vi "Read Variable (Boolean).vi"(8 "error in":errorcluster, 10 "variable name":string, 11 "particle reference in":T1) -> (0 "error out":errorcluster, 2 "value":bool, 3 "particle reference out":T1)   [LabVIEW 2013, in "Particle API.lvlib"]
doc: "Reads Spark registered variables and converts them to the relevant type (bool)."
uses:
  Particle API.lvlib
  Controls/Particle Reference.ctl
  <vilib>/httpClient/ClientHandle.ctl
  Controls/Device Query JSON.ctl
  <vilib>/httpClient/LabVIEWHTTPClient.lvlib
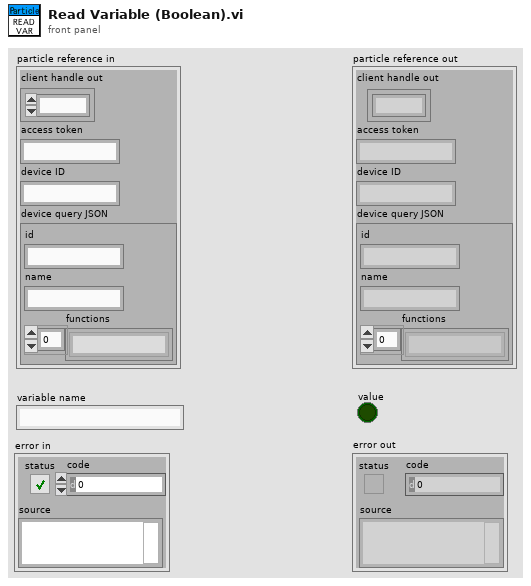
[diagram p1: front panel]
types:
  T1 = typedef "Particle API.lvlib/Particle Reference.ctl" = cluster{"client handle out":T2, "access token":string, "device ID":string, "device query JSON":T3}
  T2 = typedef "LabVIEWHTTPClient.lvlib/ClientHandle.ctl" = refnum<k1>
  T3 = typedef "Particle API.lvlib/Device Query JSON.ctl" = cluster{"id":string, "name":string, "functions":string[]}
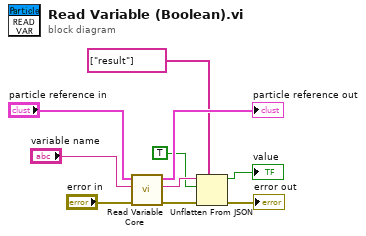
[diagram p0: block diagram]
diagram:
  n1 = call "Read Variable Core.vi"("error in"="error in", "variable name"="variable name", "particle reference in"="particle reference in") -> ("error out"=w5:errorcluster, "variable response"=w3:string, "particle reference out"=→"particle reference out":T1)  [unwired: 6 in]
  n2 = Unflatten From JSON(path=string[] ["result"], JSON string=w3, type and defaults=TRUE, error in (no error)=w5) -> (value=→"value":bool, error out=→"error out":errorcluster)  [unwired: 3 in]
